vi "savetiffs.vi"(0 "current average":sgl) -> ()   [LabVIEW 2015]
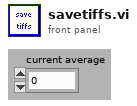
[diagram p1: front panel]
types:
  T1 = typedef "LVRectTypeDef.ctl" = cluster{"Left":i16, "Top":i16, "Right":i16, "Bottom":i16}
  T2 = cluster{"Xpixels":i32, "Vxminref":dbl, "Vxmaxref":dbl, "P":dbl, "Ypixels":i32, "Vyminref":dbl, "Vymaxref":dbl, "srate":sgl, "sAOxy":i32, "timeout":dbl, "type":string, "date":string, "time":string, "Colormap":u16, "Drawing Mode":u16, "Scanning Mode":u16, "square pixels":bool, "square matrix":bool, "Xpixels Img":i32, "Vx-min Img":dbl, "VX-max Img":dbl, "Ypixels Img":i32, "Vy-min Img":dbl, "Vy-max Img ":dbl, "Angle Img":dbl, "autoshutter":bool, "finite":bool, "cont":bool, "wavdet":bool, "measpoints":i32, "avpp":i32, "bufferAO":i32, "bufferAI":i32, "starttick":u32, "waveform":path, "Vx-ref":dbl, "Vy-ref":dbl, "refreshrate":dbl, "refreshbuffer":i32, "tt_cycles":i32, "motorref":refnum<k7>, "mirrorswitch":refnum<k7>, "sample mode":i32, "maxbufferAI":i32, "srateAODO":sgl, "bin":sgl, "Pel":sgl, "Angle draw":dbl, "srate Img":sgl, "ROIimg_plotbounds":T1, "auto OD":bool, "ODfilt":u16, "aAI":i32[], "aCI":i32[], "aAO":u32[], "aDO":u32[], "refwfsize":dbl, "Lifetime":bool, "Vz-Img":dbl, "Vz-ref":dbl, "Vz-reset":dbl, "AIoverride":bool, "aAS":u32[], "XYZstart":dbl[], "External 100KHz Clock?":bool}
  T3 = cluster{"filetif":refnum<file>[], "E_filetif":errorcluster[]}
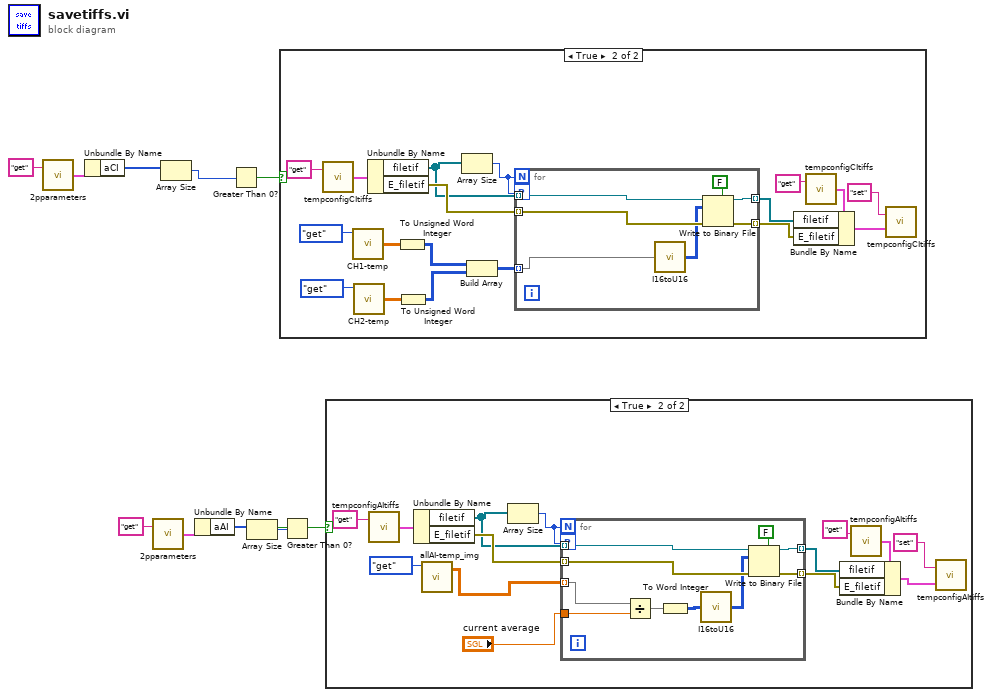
[diagram p0: block diagram]
diagram:
  n1 = call "2pparameters.vi"("command"="get") -> ("params out"=w4:T2)  [unwired: 1 in]
  n2 = Unbundle By Name(w4) -> ("aCI"=w5:i32[])
  n3 = call "2pparameters.vi"("command"="get") -> ("params out"=w9:T2)  [unwired: 1 in]
  n4 = Array Size(array=w5) -> (size(s)=w2:i32)
  n5 = Unbundle By Name(w9) -> ("aAI"=w8:i32[])
  n6 = Greater Than 0?(x=w2) -> (x > 0?=w1:bool)
  n7 = Array Size(array=w8) -> (size(s)=w7:i32)
  n8 = case shown="True" w1 {
    frame False {
    }
    frame True {
      n9 = call "tempconfigCItiffs.vi"("command"="get") -> ("Temp Config out"=w27:T3)  [unwired: 1 in]
      n10 = call "CH1-temp.vi"("command"=enum16{"get", "set", "clear", "add row"}."get") -> ("array out"=w13:sgl[][])  [unwired: 3 in, 1 out]
      n11 = call "CH2-temp.vi"("command"=enum16{"get", "set", "clear", "add row"}."get") -> ("array out"=w14:sgl[][])  [unwired: 3 in, 1 out]
      n12 = Unbundle By Name(w27) -> ("filetif"=w23:refnum<file>[], "E_filetif"=w28:errorcluster[])
      n13 = To Unsigned Word Integer(number=w13) -> (unsigned 16bit integer=w16:u16[][])
      n14 = To Unsigned Word Integer(number=w14) -> (unsigned 16bit integer=w17:u16[][])
      n15 = Array Size(array=w23) -> (size(s)=w22:i32)
      n16 = Build Array(w16, w17) -> (w11:u16[][][])
      n17 = for {
        N: w22 -> [_]
        tunnel: w28 -> [w35] mode=indexing
        tunnel: w23 -> [w34] mode=indexing
        tunnel: [w32] -> w25 mode=indexing
        tunnel: [w31] -> w24 mode=indexing
        workers-P: w22 -> [_]
        tunnel: w11 -> [w29] mode=indexing
        n18 = call "I16toU16.vi"("I16"=w29) -> ("U16"=w30:u16[][])
        n19 = Write to Binary File(file (use dialog)=w34, data=w30, error in=w35, 5:FALSE ("prepend array or string size? (T)")) -> (refnum out=w32:refnum<file>, error out=w31:errorcluster)  [unwired: 2 in, 1 out]
      }
      n20 = call "tempconfigCItiffs.vi"("command"="get") -> ("Temp Config out"=w19:T3)  [unwired: 1 in]
      n21 = Bundle By Name(cluster=w19, "filetif"=w25, "E_filetif"=w24) -> (w21:T3)
      n22 = call "tempconfigCItiffs.vi"("Temp Config in"=w21, "command"="set") -> ()  [unwired: 1 out]
    }
  }
  n23 = Greater Than 0?(x=w7) -> (x > 0?=w6:bool)
  n24 = case shown="True" w6 {
    frame False {
    }
    frame True {
      n25 = call "tempconfigAItiffs.vi"("command"="get") -> ("Temp Config out"=w48:T3)  [unwired: 1 in]
      n26 = Unbundle By Name(w48) -> ("filetif"=w39:refnum<file>[], "E_filetif"=w49:errorcluster[])
      n27 = call "allAI-temp_img.vi"("command"=enum16{"get", "set", "clear", "append"}."get") -> ("array out"=w36:sgl[][][])  [unwired: 3 in, 1 out]
      n28 = Array Size(array=w39) -> (size(s)=w38:i32)
      n29 = for {
        N: w38 -> [_]
        tunnel: w49 -> [w59] mode=indexing
        tunnel: w39 -> [w58] mode=indexing
        tunnel: [w56] -> w44 mode=indexing
        tunnel: [w55] -> w43 mode=indexing
        tunnel: w36 -> [w50] mode=indexing
        workers-P: w38 -> [_]
        tunnel: "current average" -> [w51]
        n30 = Divide(x=w50, y=w51) -> (x/y=w54:sgl[][])
        n31 = To Word Integer(number=w54) -> (16bit integer=w53:i16[][])
        n32 = call "I16toU16.vi"("I16"=w53) -> ("U16"=w52:u16[][])
        n33 = Write to Binary File(file (use dialog)=w58, data=w52, error in=w59, 5:FALSE ("prepend array or string size? (T)")) -> (refnum out=w56:refnum<file>, error out=w55:errorcluster)  [unwired: 2 in, 1 out]
      }
      n34 = call "tempconfigAItiffs.vi"("command"="get") -> ("Temp Config out"=w45:T3)  [unwired: 1 in]
      n35 = Bundle By Name(cluster=w45, "filetif"=w44, "E_filetif"=w43) -> (w40:T3)
      n36 = call "tempconfigAItiffs.vi"("Temp Config in"=w40, "command"="set") -> ()  [unwired: 1 out]
    }
  }
